vi "SetActiveData_LoadedFromVI.vi"(7 "Layer Template":refnum<vi>, 8 "error in (no error)":errorcluster, 9 "Match?":bool, 10 "Match Index":i32, 11 "FakedArray in":refnum<class "FakedArray.lvclass">) -> (0 "error out":errorcluster, 2 "Position Scrollbar":i32, 3 "FakedArray out":refnum<class "FakedArray.lvclass">, 5 "Valid?":bool)   [LabVIEW 2021, in "FakedArray.lvclass"]
uses:
  <resource>/plugins/NIIconEditor/Class/FakedArray/FakedArray.lvclass
  <vilib>/LabVIEW Icon API/lv_icon/Controls/Graphic.ctl
  <vilib>/LabVIEW Icon API/lv_icon/Controls/Layer.ctl
  <resource>/plugins/NIIconEditor/Class/FakedArray/FakedArray.lvclass/FakedArray.ctl
  <vilib>/LabVIEW Icon API/lv_icon/Controls/Pathes.ctl
  <vilib>/LabVIEW Icon API/lv_icon/lv_icon.lvlib
panel:
  in  "Filter":string="LabVIEW Icon API"
  in  "?":T1
  in  "?":T1
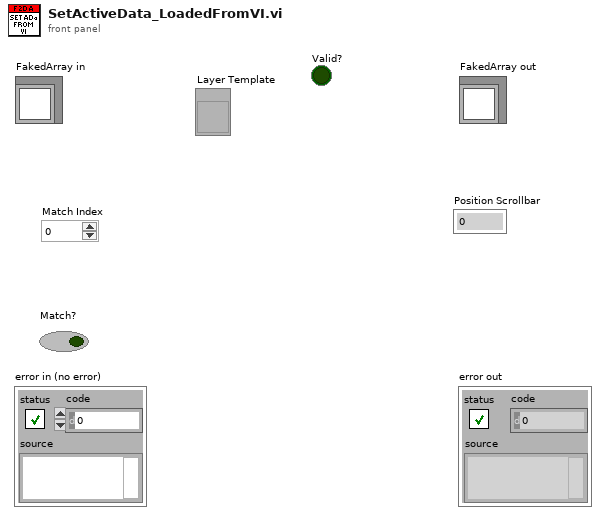
[diagram p1: front panel]
types:
  T1 = typedef "Graphic.ctl" = cluster{"Rectangle":cluster{"left":i16, "top":i16, "right":i16, "bottom":i16}, "Path":path, "Image":picture, "Filter":string, "FileName":string}
  T2 = typedef "Layer.ctl" = cluster{"LayerIcon":picture, "LayerName":string, "Opacity":u8, "Visibility?":bool}
  T3 = enum32{"Unknown Icon Source", "VI Icon", "Library Icon (any library type)", "Palette icon", "Icon from App Method"}
  T4 = typedef "Pathes.ctl" = enum16{"Root Path", "Icon Templates", "Icon Templates VI", "Icon Templates Lib", "Glyphs"}
  T5 = cluster{"left":i16, "top":i16, "right":i16, "bottom":i16}
  T6 = typedef "Icon Editor Invoker Type.ctl" = enum32{"Unknown Icon Source", "VI Icon", "Library Icon (any library type)", "Palette icon", "Icon from App Method"}
  T7 = typedef "LabVIEW Icon Stored Information.ctl" = cluster{"Text Visible?":bool, "Text Opacity":u8, "Templ Visible?":bool, "Templ Opacity":u8, "Relative Path from 1 to 2":path, "Image":picture, "All User Layers":refnum<class "Layer.lvclass">[], "Body Text":T8}
  T8 = typedef "BodyText.ctl" = cluster{"Line 1 text":string, "Line 2 text":string, "Line 3 text":string, "Line 4 text":string, "Line 1 color":u32, "Line 2 color":u32, "Line 3 color":u32, "Line 4 color":u32, "Body Text Spec":cluster{"Font":T9, "Alignment":T10, "Size":u8}, "Center text vertically":bool, "Capitalize Text":bool}
  T9 = typedef "Font.ctl" = string
  T10 = typedef "Alignment.ctl" = u16
  T11 = cluster{"LayerIcon":picture, "LayerName":string, "Opacity":u8, "Visibility?":bool}
  T12 = typedef "INI.ctl" = cluster{"Show Layer Tab?":bool, "Show Terminals?":bool, "Text":cluster{"Font":T9, "Alignment":T10, "Size":T13}, "3rd party Templates":cluster{"Store 3rd party Templates?":bool, "Folder Name":string}, "Merge user layers on commit":bool, "Body Text":T8, "Fill Color":T14, "Edge Color":T14, "Tab":u16, "Tool":T15, "Disable Layers?":bool}
  T13 = typedef "Font Size.ctl" = u8
  T14 = typedef "IEColor.ctl" = u32
  T15 = typedef "Tools.ctl" = enum32{"Pencil", "Line", "Dropper", "Fill", "Rectangle", "Filled Rectangle", "Ellipse", "Filled Ellipse", "Eraser", "Text", "Select", "Move"}
  T16 = typedef "imagedata.ctl" = cluster{"image type":i32, "image depth":i32, "image":u8[], "mask":u8[], "colors":u32[], "Rectangle":cluster{"left":i16, "top":i16, "right":i16, "bottom":i16}}
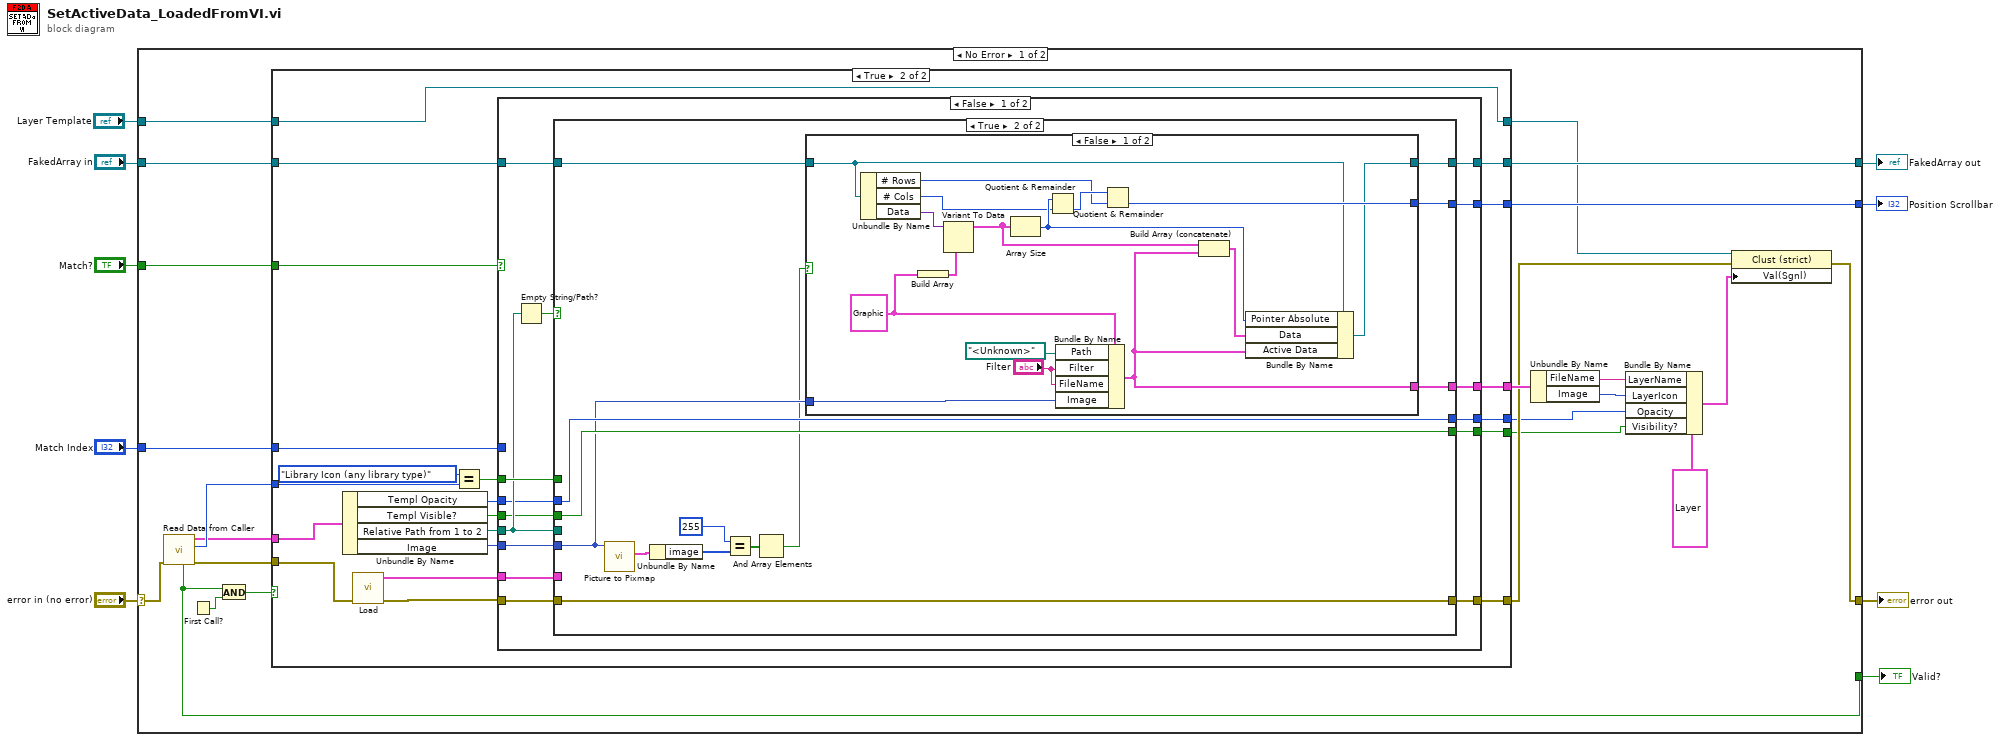
[diagram p0: block diagram]
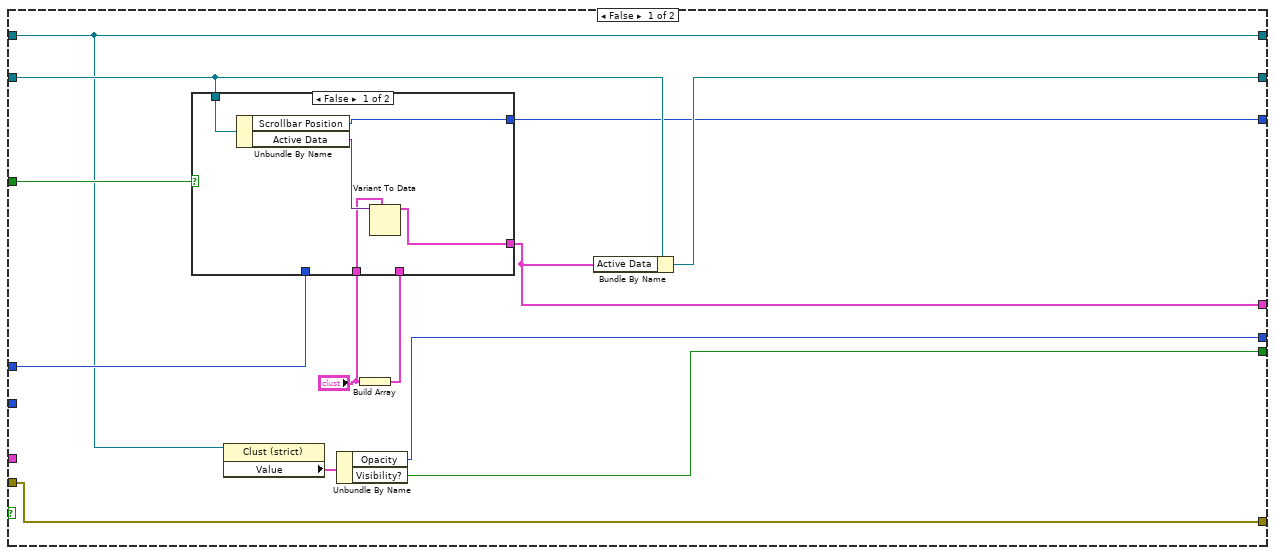
[diagram p2: hidden frame]
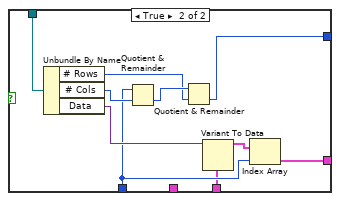
[diagram p3: hidden frame]
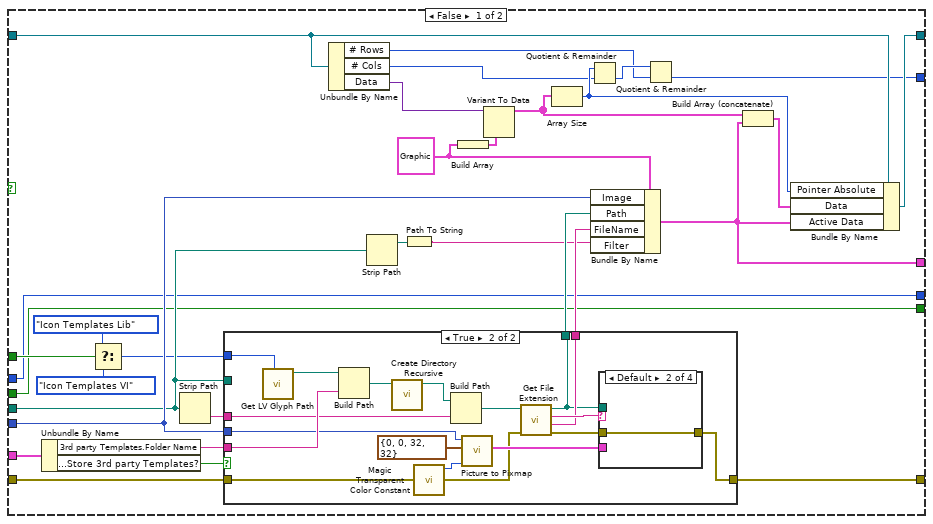
[diagram p4: hidden frame]
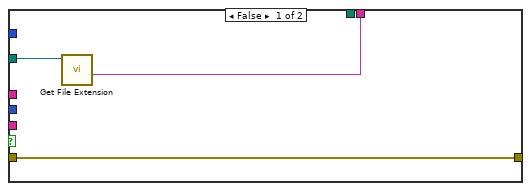
[diagram p5: hidden frame]
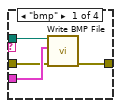
[diagram p6: hidden frame]
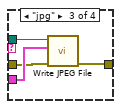
[diagram p7: hidden frame]
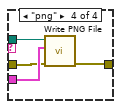
[diagram p8: hidden frame]
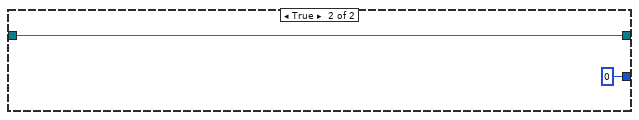
[diagram p9: hidden frame]
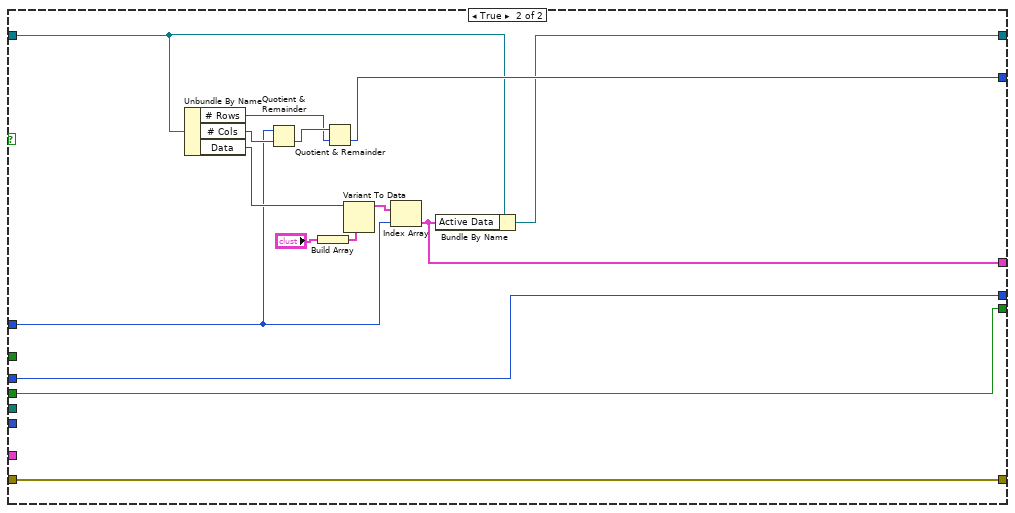
[diagram p10: hidden frame]
diagram:
  n1 = case shown="No Error" "error in (no error)" {
    selector: "error in (no error)" -> [w30 w208]
    tunnel: [w19 w208] -> w8
    tunnel: [w31 w207] -> w6
    tunnel: "FakedArray in" -> [w32 w207]
    tunnel: "Match Index" -> [w27 _]
    tunnel: "Match?" -> [w28 _]
    tunnel: [w26 _] -> w3
    tunnel: [w18 _] -> w2
    tunnel: "Layer Template" -> [w11 _]
    frame No Error {
      n2 = call <resource>:"Read Data from Caller.vi"("error in (no error)"=w30) -> ("error out"=w29:errorcluster, "Icon Editor Invoker Type"=w25:T6, "data"=w12:T7, "Valid?"=w18:bool)  [unwired: 2 in, 5 out]
      n3 = First Call?() -> (First Call?: T/F=w17:bool)
      n4 = And(x=w18, y=w17) -> (x .and. y?=w16:bool)
      n5 = case shown="True" w16 {
        tunnel: w32 -> [w44 w80]
        tunnel: [w43 w74] -> w31
        tunnel: w12 -> [_ w81]
        tunnel: w29 -> [w45 w77]
        tunnel: w28 -> [w39 w79]
        tunnel: w27 -> [w42 w76]
        tunnel: [w45 w75] -> w15
        tunnel: [w41 w73] -> w26
        tunnel: w25 -> [_ w69]
        tunnel: [w40 w66] -> w24
        tunnel: [w34 w63] -> w14
        tunnel: [w33 w62] -> w13
        tunnel: w11 -> [w36 w61]
        tunnel: [w36 w61] -> w10
        frame False {
          n6 = property class="Clust (strict)"(reference=w36) -> ("Value"=w35:T11)  [unwired: 1 in, 2 out]
          n7 = Unbundle By Name(w35) -> ("Opacity"=w34:u8, "Visibility?"=w33:bool)
          n8 = Build Array("?") -> (w38:T1[])
          n9 = case shown="False" w39 {
            tunnel: w44 -> [w50 w55]
            tunnel: w42 -> [_ w54]
            tunnel: [w49 w53] -> w41
            tunnel: [w46 w52] -> w40
            tunnel: w38 -> [_ w51]
            tunnel: "?" -> [w47 _]
            frame False {
              n10 = Unbundle By Name(w50) -> ("Scrollbar Position"=w49:i32, "Active Data"=w48:variant)
              n11 = Variant To Data(type=w47, Variant=w48) -> (data=w46:T1)  [unwired: 1 in, 1 out]
            }
            frame True {
              n12 = Unbundle By Name(w55) -> ("# Rows"=w58:i32, "# Cols"=w59:i32, "Data"=w57:variant)
              n13 = Quotient & Remainder(x=w54, y=w59) -> (floor(x/y)=w60:i32)  [unwired: 1 out]
              n14 = Quotient & Remainder(x=w60, y=w58) -> (floor(x/y)=w53:i32)  [unwired: 1 out]
              n15 = Variant To Data(type=w51, Variant=w57) -> (data=w56:T1[])  [unwired: 1 in, 1 out]
              n16 = Index Array(array=w56, index=w54) -> (element=w52:T1)
            }
          }
          n17 = Bundle By Name(cluster=w44, "Active Data"=w40) -> (w43:refnum<class "FakedArray.lvclass">)
        }
        frame True {
          n18 = Unbundle By Name(w81) -> ("Templ Opacity"=w64:u8, "Templ Visible?"=w65:bool, "Relative Path from 1 to 2"=w78:path, "Image"=w70:picture)
          n19 = call <resource>:"Load.vi"("error in"=w77) -> ("error out"=w71:errorcluster, "INI Data"=w72:T12)  [unwired: 1 in, 8 out]
          n20 = Equal?(x=T3."Library Icon (any library type)", y=w69) -> (x = y?=w67:bool)
          n21 = case shown="False" w79 {
            tunnel: w80 -> [w92 w198]
            tunnel: w78 -> [w87 _]
            tunnel: w72 -> [w96 _]
            tunnel: w71 -> [w95 w206]
            tunnel: [w94 w206] -> w75
            tunnel: w76 -> [_ w196]
            tunnel: [w93 w197] -> w74
            tunnel: [w91 w202] -> w73
            tunnel: w70 -> [w90 _]
            tunnel: w67 -> [w89 _]
            tunnel: [w88 w194] -> w66
            tunnel: w65 -> [w85 w192]
            tunnel: w64 -> [w84 w193]
            tunnel: [w83 w193] -> w63
            tunnel: [w82 w192] -> w62
            frame False {
              n22 = Empty String/Path?(string/path=w87) -> (empty?=w86:bool)
              n23 = case shown="True" w86 {
                tunnel: w96 -> [w127 _]
                tunnel: w95 -> [w126 w173]
                tunnel: [w125 w173] -> w94
                tunnel: [w124 w167] -> w93
                tunnel: w92 -> [w123 w168]
                tunnel: [w115 w169] -> w91
                tunnel: w90 -> [w112 w166]
                tunnel: w89 -> [w111 _]
                tunnel: [w110 w170] -> w88
                tunnel: w87 -> [w109 _]
                tunnel: w85 -> [w97 w171]
                tunnel: w84 -> [w98 w172]
                tunnel: [w98 w172] -> w83
                tunnel: [w97 w171] -> w82
                frame False {
                  w114 = T1 {"Rectangle"={"left"=0, "top"=0, "right"=0, "bottom"=0}, "Path"=path "", "Image"=bytes[0], "Filter"="", "FileName"=""}
                  n24 = Unbundle By Name(w127) -> ("3rd party Templates.Folder Name"=w108:string, "3rd party Templates.Store 3rd party Templates?"=w106:bool)
                  n25 = Select(t=Pathes."Icon Templates Lib" ("Path"), s=w111, f=Pathes."Icon Templates VI" ("Path")) -> (s? t:f=w101:T4)
                  n26 = Strip Path(path=w109) -> (name=w104:string)  [unwired: 1 out]
                  n27 = case shown="True" w106 {
                    tunnel: w108 -> [_ w146]
                    tunnel: w126 -> [w129 w141]
                    tunnel: [w129 w139] -> w125
                    tunnel: [w130 w137] -> w107
                    tunnel: w112 -> [_ w136]
                    tunnel: [_ w134] -> w105
                    tunnel: w104 -> [_ w133]
                    tunnel: w109 -> [w128 _]
                    tunnel: w101 -> [_ w132]
                    frame False {
                      n28 = call <vilib>:"Get File Extension.vi"("file"=w128) -> ("filename without extension"=w130:string)  [unwired: 1 in, 9 out]
                    }
                    frame True {
                      n29 = call <vilib>:"Get LV Glyph Path.vi"("Path"=w132) -> ("Requested Path"=w147:path)  [unwired: 2 in, 8 out]
                      n30 = Build Path(base path=w147, name or relative path=w146) -> (appended path=w135:path)
                      n31 = call <vilib>:"Create Directory Recursive.vi"("directory"=w135) -> ("directory copy"=w144:path)  [unwired: 2 in, 4 out]
                      n32 = call <vilib>:"Magic Transparent Color Constant.vi"() -> ("Magic transparent color constant"=w131:u32)  [unwired: 11 out]
                      n33 = Build Path(base path=w144, name or relative path=w133) -> (appended path=w138:path)
                      n34 = call <vilib>:"Picture to Pixmap.vi"("Background Color"=w131, "rect"=T5 {"left"=0, "top"=0, "right"=32, "bottom"=32}, "picture"=w136) -> ("image data"=w142:T16)  [unwired: 1 in, 7 out]
                      n35 = call <vilib>:"Get File Extension.vi"("error in (no error)"=w141, "file"=w138) -> ("error out"=w140:errorcluster, "filename without extension"=w137:string, "lowercase file extension"=w143:string, "dup file"=w134:path)  [unwired: 6 out]
                      n36 = case shown="Default" w143 {
                        tunnel: w134 -> [w151 _ w156 w160]
                        tunnel: w142 -> [w150 _ w155 w159]
                        tunnel: w140 -> [w149 w152 w154 w158]
                        tunnel: [w148 w152 w153 w157] -> w139
                        frame "bmp" {
                          n37 = call <vilib>:"Write BMP File.vi"("error in (no error)"=w149, "image data"=w150, "path to BMP file"=w151) -> ("error out"=w148:errorcluster)  [unwired: 8 out]
                        }
                        frame Default {
                        }
                        frame "jpg" {
                          n38 = call <vilib>:"Write JPEG File.vi"("error in (no error)"=w154, "image data"=w155, "path to JPEG file"=w156) -> ("error out"=w153:errorcluster)  [unwired: 8 out]
                        }
                        frame "png" {
                          n39 = call <vilib>:"Write PNG File.vi"("error in (no error)"=w158, "image data"=w159, "path to PNG file"=w160) -> ("error out"=w157:errorcluster)  [unwired: 8 out]
                        }
                      }
                    }
                  }
                  n40 = Unbundle By Name(w123) -> ("# Rows"=w116:i32, "# Cols"=w118:i32, "Data"=w122:variant)
                  n41 = Strip Path(path=w109) -> (stripped path=w100:path)  [unwired: 1 out]
                  n42 = Path To String(path=w100) -> (string=w99:string)
                  n43 = Build Array(w114) -> (w113:T1[])
                  n44 = Variant To Data(type=w113, Variant=w122) -> (data=w120:T1[])  [unwired: 1 in, 1 out]
                  n45 = Array Size(array=w120) -> (size(s)=w119:i32)
                  n46 = Quotient & Remainder(x=w119, y=w118) -> (floor(x/y)=w117:i32)  [unwired: 1 out]
                  n47 = Bundle By Name(cluster=w114, "Image"=w112, "Path"=w105, "FileName"=w107, "Filter"=w99) -> (w110:T1)
                  n48 = Quotient & Remainder(x=w117, y=w116) -> (floor(x/y)=w115:i32)  [unwired: 1 out]
                  n49 = Build Array (concatenate)(w120, w110) -> (w121:T1[])
                  n50 = Bundle By Name(cluster=w123, "Pointer Absolute"=w119, "Data"=w121, "Active Data"=w110) -> (w124:refnum<class "FakedArray.lvclass">)
                }
                frame True {
                  n51 = call <vilib>:"Picture to Pixmap.vi"("picture"=w166) -> ("image data"=w165:T16)  [unwired: 9 in, 1 out]
                  n52 = Unbundle By Name(w165) -> ("image"=w164:u8[])
                  n53 = Equal?(x=u8 255, y=w164) -> (x = y?=w162:bool[])
                  n54 = And Array Elements(Boolean array=w162) -> (logical AND=w161:bool)
                  n55 = case shown="False" w161 {
                    tunnel: [w178 _] -> w170
                    tunnel: [w177 0] -> w169
                    tunnel: w168 -> [w176 w191]
                    tunnel: [w175 w191] -> w167
                    tunnel: w166 -> [w174 _]
                    frame False {
                      w179 = T1 {"Rectangle"={"left"=0, "top"=0, "right"=0, "bottom"=0}, "Path"=path "", "Image"=bytes[0], "Filter"="", "FileName"=""}
                      # "Localized"
                      n56 = Unbundle By Name(w176) -> ("# Rows"=w182:i32, "# Cols"=w184:i32, "Data"=w188:variant)
                      n57 = Build Array(w179) -> (w181:T1[])
                      n58 = Variant To Data(type=w181, Variant=w188) -> (data=w186:T1[])  [unwired: 1 in, 1 out]
                      n59 = Array Size(array=w186) -> (size(s)=w185:i32)
                      n60 = Quotient & Remainder(x=w185, y=w184) -> (floor(x/y)=w183:i32)  [unwired: 1 out]
                      n61 = Bundle By Name(cluster=w179, "Path"=path "<Unknown>", "Filter"="Filter", "FileName"="Filter", "Image"=w174) -> (w178:T1)
                      n62 = Quotient & Remainder(x=w183, y=w182) -> (floor(x/y)=w177:i32)  [unwired: 1 out]
                      n63 = Build Array (concatenate)(w186, w178) -> (w187:T1[])
                      n64 = Bundle By Name(cluster=w176, "Pointer Absolute"=w185, "Data"=w187, "Active Data"=w178) -> (w175:refnum<class "FakedArray.lvclass">)
                    }
                    frame True {
                    }
                  }
                }
              }
            }
            frame True {
              n65 = Unbundle By Name(w198) -> ("# Rows"=w203:i32, "# Cols"=w204:i32, "Data"=w199:variant)
              n66 = Quotient & Remainder(x=w196, y=w204) -> (floor(x/y)=w205:i32)  [unwired: 1 out]
              n67 = Build Array("?") -> (w200:T1[])
              n68 = Quotient & Remainder(x=w205, y=w203) -> (floor(x/y)=w202:i32)  [unwired: 1 out]
              n69 = Variant To Data(type=w200, Variant=w199) -> (data=w195:T1[])  [unwired: 1 in, 1 out]
              n70 = Index Array(array=w195, index=w196) -> (element=w194:T1)
              n71 = Bundle By Name(cluster=w198, "Active Data"=w194) -> (w197:refnum<class "FakedArray.lvclass">)
            }
          }
        }
      }
      n72 = Unbundle By Name(w24) -> ("FileName"=w22:string, "Image"=w21:picture)
      n73 = Bundle By Name(cluster=T2 {"LayerIcon"=bytes[0], "LayerName"="", "Opacity"=0, "Visibility?"=FALSE}, "LayerName"=w22, "LayerIcon"=w21, "Opacity"=w14, "Visibility?"=w13) -> (w20:T2)
      n74 = property class="Clust (strict)"(reference=w10, error in=w15, "Val(Sgnl)"=w20) -> (error out=w19:errorcluster)  [unwired: 1 out]
    }
    frame Error {
    }
  }
  "error out" <- w8
  "FakedArray out" <- w6
  "Position Scrollbar" <- w3
  "Valid?" <- w2
